vi "sampling.vi"() -> ()   [LabVIEW 2020, in "I2C Module.lvlib"]
uses:
  I2C Module.lvlib
panel:
  out "nearest frequency":dbl
  in  "sample rate":dbl=1000.0 format="%0.2f"
  in  "samples":dbl=1000.0
  in  "frequency":dbl=100.0 format="%0.2f"
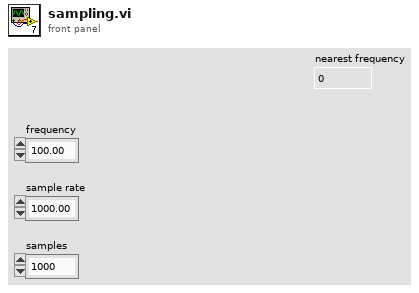
[diagram p1: front panel]
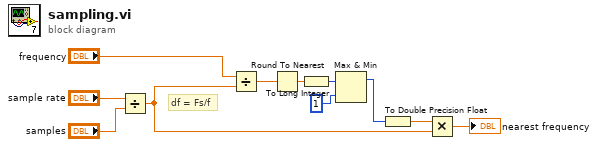
[diagram p0: block diagram]
diagram:
  # "df = Fs/f"
  n1 = Divide(x="sample rate", y="samples") -> (x/y=w9:dbl)
  n2 = Divide(x="frequency", y=w9) -> (x/y=w6:dbl)
  n3 = Round To Nearest(number=w6) -> (nearest integer value=w10:dbl)
  n4 = To Long Integer(number=w10) -> (32bit integer=w5:i32)
  n5 = Max & Min(x=w5, y=1) -> (max(x,y)=w4:i32)  [unwired: 1 out]
  n6 = To Double Precision Float(number=w4) -> (double precision float=w3:dbl)
  n7 = Multiply(x=w3, y=w9) -> (x*y=→"nearest frequency":dbl)
